vi "ProductRequest.vi"(8 "error in (no error)":errorcluster, 10 "Product Index":i32, 11 "Prooduct Actor in":refnum<class "Prooduct Actor.lvclass">) -> (0 "error out":errorcluster, 3 "Prooduct Actor out":refnum<class "Prooduct Actor.lvclass">)   [LabVIEW 2020, in "Prooduct Actor.lvlib" / "Prooduct Actor.lvclass"]
uses:
  Prooduct Actor.lvclass
  C:/Program Files (x86)/National Instruments/LabVIEW 2020/vi.lib/ActorFramework/Actor/Actor.lvclass
  <vilib>/ActorFramework/Actor/Actor.lvclass/Actor.ctl
  Prooduct Actor.lvclass/Prooduct Actor.ctl
  UI Actor Messages/ProductRequest Msg/ProductRequest Msg.lvclass/ProductRequest Msg.ctl
  <vilib>/ActorFramework/Message Enqueuer/Message Enqueuer.lvclass/Message Enqueuer.ctl
  <vilib>/ActorFramework/Message Enqueuer/Enqueue.vi
  UI Actor Messages/ProductRequest Msg/ProductRequest Msg.lvclass
  C:/Program Files (x86)/National Instruments/LabVIEW 2020/vi.lib/ActorFramework/Message/Message.lvclass
  <vilib>/ActorFramework/Message Priority Queue/Priority Enqueue.vi
  <vilib>/ActorFramework/Actor/Actor.lvclass
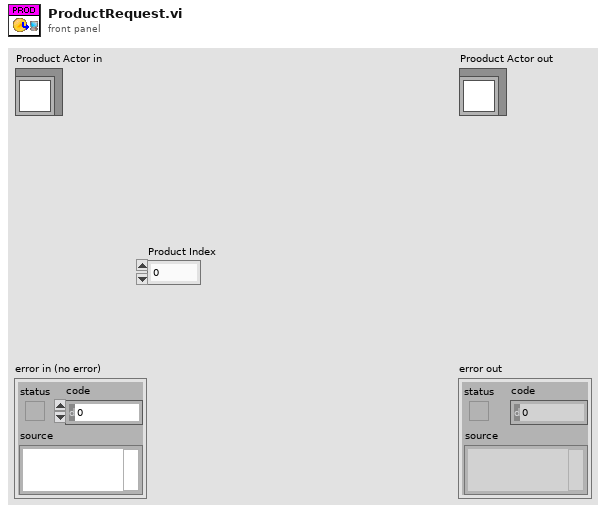
[diagram p1: front panel]
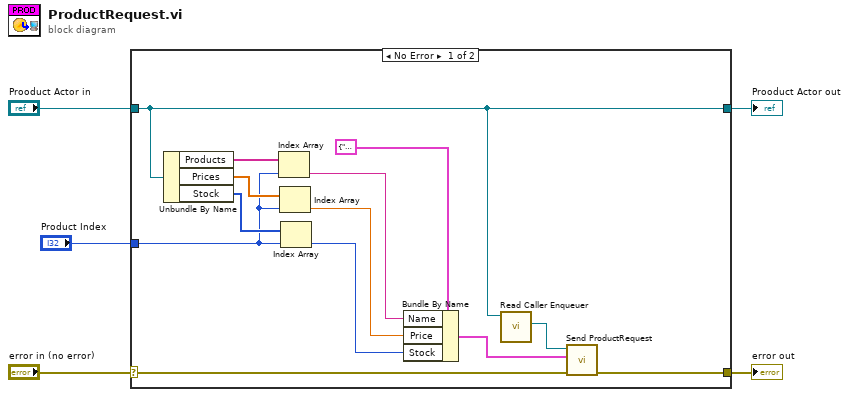
[diagram p0: block diagram]
diagram:
  n1 = case shown="No Error" "error in (no error)" {
    selector: "error in (no error)" -> [w18 w20]
    tunnel: [w17 w20] -> w4
    tunnel: [w15 w19] -> w2
    tunnel: "Prooduct Actor in" -> [w15 w19]
    tunnel: "Product Index" -> [w11 _]
    frame No Error {
      n2 = Unbundle By Name(w15) -> ("Products"=w14:string[], "Prices"=w13:dbl[], "Stock"=w12:i32[])
      n3 = Index Array(array=w14, index=w11) -> (element=w8:string)
      n4 = Index Array(array=w13, index=w11) -> (element=w7:dbl)
      n5 = Index Array(array=w12, index=w11) -> (element=w6:i32)
      n6 = Bundle By Name(cluster=cluster{"Name":string, "Price":dbl, "Stock":i32} {"Name"="", "Price"=0.0, "Stock"=0} ("Product Info"), "Name"=w8, "Price"=w7, "Stock"=w6) -> (w9:cluster{"Name":string, "Price":dbl, "Stock":i32})
      n7 = call <vilib>:"Read Caller Enqueuer.vi"("Actor"=w15) -> ("Caller Enqueuer"=w16:refnum<class "Message Enqueuer.lvclass">)  [unwired: 10 in]
      n8 = call "Send ProductRequest.vi"("error in (no error)"=w18, "Product Info"=w9, "Message Enqueuer"=w16) -> ("error out"=w17:errorcluster)  [unwired: 7 in, 1 out]
    }
    frame Error {
    }
  }
  "error out" <- w4
  "Prooduct Actor out" <- w2
